vi "_Open Sequence File.vi"(7 "Load Options":T1={"Use Search Dirs? (T)"=TRUE, "Conflict as Error? (T)"=TRUE, "Check Station Model? (F)"=FALSE, "Preload Modules? (T)"=TRUE, "Skip Load Callback? (F)"=FALSE, "Reload if Loaded? (F)"=FALSE}, 8 "error in (no error)":errorcluster, 9 "Current Seq File (None)":T2, 10 "File Path":string, 11 "Engine in":refnum<class "Engine.lvclass">) -> (0 "error out":errorcluster, 2 "SeqFile Ref":refnum<k7>, 3 "Engine out":refnum<class "Engine.lvclass">)   [LabVIEW 2020, in "TSS.lvlib" / "Engine.lvclass"]
uses:
  Engine.lvclass
  SequenceFile/Typedefs/Session Handle.ctl
  SequenceFile/SequenceFile.lvclass
  Data Types/File Load Options.ctl
  Engine.lvclass/Engine.ctl
  TSS.lvlib
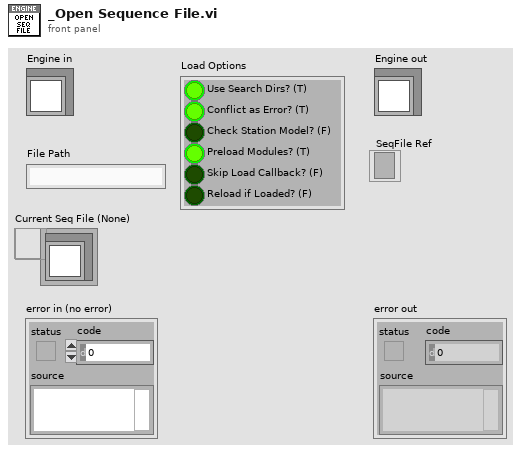
[diagram p1: front panel]
types:
  T1 = typedef "TSS.lvlib/File Load Options.ctl" = cluster{"Use Search Dirs? (T)":bool, "Conflict as Error? (T)":bool, "Check Station Model? (F)":bool, "Preload Modules? (T)":bool, "Skip Load Callback? (F)":bool, "Reload if Loaded? (F)":bool}
  T2 = typedef "TSS.lvlib/SequenceFile.lvclass/Session Handle.ctl" = refnum<data-value>
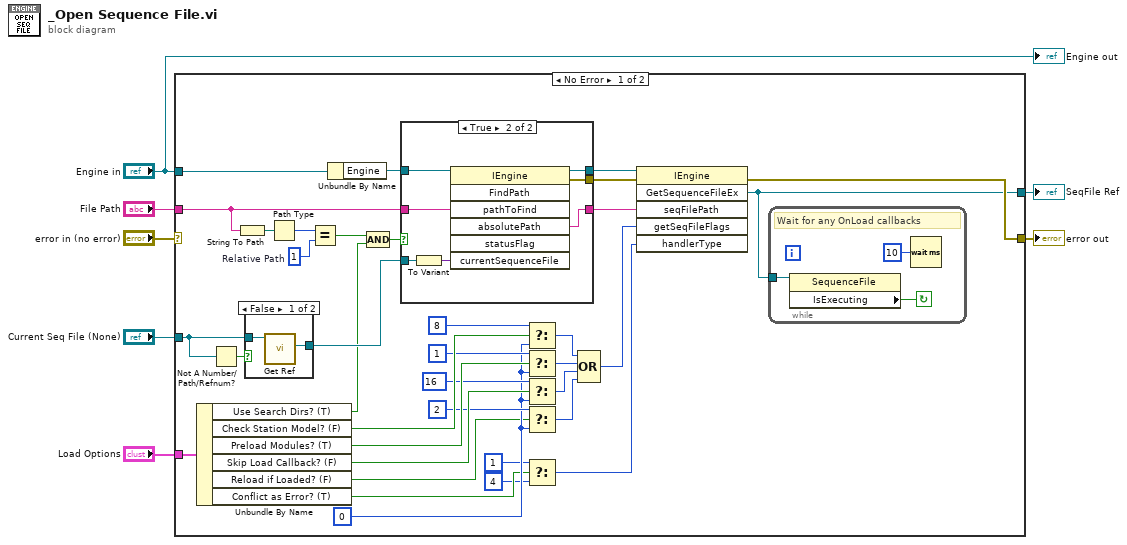
[diagram p0: block diagram]
diagram:
  n1 = case shown="No Error" "error in (no error)" {
    selector: "error in (no error)" -> [_ w58]
    tunnel: "Engine in" -> [w42 _]
    tunnel: "File Path" -> [w35 _]
    tunnel: "Current Seq File (None)" -> [w32 _]
    tunnel: "Load Options" -> [w29 _]
    tunnel: [w43 w58] -> w4
    tunnel: [w8 _] -> w2
    frame No Error {
      w20 = 0 ("getSeqFileFlags")
      w38 = i16 1  # Relative Path
      n2 = Unbundle By Name(w29) -> ("Use Search Dirs? (T)"=w28:bool, "Check Station Model? (F)"=w27:bool, "Preload Modules? (T)"=w25:bool, "Skip Load Callback? (F)"=w22:bool, "Reload if Loaded? (F)"=w19:bool, "Conflict as Error? (T)"=w17:bool)
      n3 = Not A Number/Path/Refnum?(number/path/refnum=w32) -> (NaN/Path/Refnum?=w33:bool)
      n4 = String To Path(string=w35) -> (path=w40:path)
      n5 = case shown="False" w33 {
        tunnel: w32 -> [w48 _]
        tunnel: [w47 _] -> w31
        frame False {
          n6 = call "Get Ref.vi"("Session Handle in"=w48) -> ("Ref"=w47:refnum<k7>)  [unwired: 8 in, 2 out]
        }
        frame True {
        }
      }
      n7 = Path Type(1:w40) -> (0:w39:i16)
      n8 = Equal?(x=w39, y=w38) -> (x = y?=w36:bool)
      n9 = Unbundle By Name(w42) -> ("Engine"=w41:refnum<k7>)
      n10 = Compound Arithmetic op=AND(w36, w28) -> (w37:bool)
      n11 = case shown="True" w37 {
        tunnel: w41 -> [w49 w57]
        tunnel: w35 -> [w50 w56]
        tunnel: [w50 w55] -> w30
        tunnel: [w49 w54] -> w34
        tunnel: w31 -> [_ w53]
        tunnel: [_ w51] -> w9
        frame False {
        }
        frame True {
          n12 = To Variant(anything=w53) -> (Variant=w52:variant)
          n13 = invoke class="IEngine" method="FindPath"(reference=w57, "pathToFind"=w56, "currentSequenceFile"=w52) -> (reference out=w54:refnum<k7>, error out=w51:errorcluster, "absolutePath"=w55:string)  [unwired: 4 in, 4 out]
        }
      }
      n14 = Select(t=8 ("getSeqFileFlags"), s=w27, f=w20) -> (s? t:f=w13:i32)
      n15 = Select(t=1 ("getSeqFileFlags"), s=w25, f=w20) -> (s? t:f=w14:i32)
      n16 = Select(t=16 ("getSeqFileFlags"), s=w22, f=w20) -> (s? t:f=w12:i32)
      n17 = Select(t=2 ("getSeqFileFlags"), s=w19, f=w20) -> (s? t:f=w11:i32)
      n18 = Select(t=1 ("getSeqFileFlags"), s=w17, f=4 ("getSeqFileFlags")) -> (s? t:f=w15:i32)
      n19 = Compound Arithmetic op=OR(w13, w14, w12, w11) -> (w10:i32)
      n20 = invoke class="IEngine" method="GetSequenceFileEx"(reference=w34, error in=w9, "seqFilePath"=w30, "getSeqFileFlags"=w10, "handlerType"=w15) -> (error out=w43:errorcluster, "GetSequenceFileEx"=w8:refnum<k7>)  [unwired: 1 in, 4 out]
      n21 = while {
        tunnel: w8 -> [w46]
        stop <- w45 continue-if-true
        # "Wait for any OnLoad callbacks"
        n22 = property class="SequenceFile"(reference=w46) -> ("IsExecuting"=w45:bool)  [unwired: 1 in, 2 out]
        n23 = Wait (ms)(milliseconds to wait=u32 10) -> ()  [unwired: 1 out]
      }
    }
    frame Error {
    }
  }
  "error out" <- w4
  "SeqFile Ref" <- w2
  "Engine out" <- "Engine in"
